vi "Test Broadcast Seen from Process Added Before Attaching to Owning Application.vi"(8 "error in (no error)":errorcluster, 11 "Test Case In":refnum<class "Monitor Broadcasts Test.lvclass">) -> (0 "error out":errorcluster, 3 "Test Case Out":refnum<class "Monitor Broadcasts Test.lvclass">)   [LabVIEW 2020, in "Monitor Broadcasts Test.lvclass"]
uses:
  Monitor Broadcasts Test.lvclass
  C:/Program Files (x86)/National Instruments/LabVIEW 2020/vi.lib/Astemes/LUnit/Test Case.lvclass
  source/Broadcast Message Receiver/Broadcast Message Receiver.lvclass
  C:/Git/astemes-triarc-debugger/source/Process/Debug Process.lvclass
  <vilib>/Astemes/Triarc Framework/Application/Application.lvclass
  C:/Program Files (x86)/National Instruments/LabVIEW 2020/vi.lib/Astemes/Triarc Framework/Process/Process.lvclass
  <vilib>/Astemes/Triarc Framework/Process/Process.lvclass
  <vilib>/Astemes/Triarc Framework/Process/Process.lvclass/Process.ctl
  <vilib>/Astemes/Triarc Framework/Application/Application.lvclass/Application.ctl
  source/Process/Debug Process.lvclass/Debug Process.ctl
  source/Broadcast Message Receiver/Broadcast Message Receiver.lvclass/Broadcast Message Receiver.ctl
  <vilib>/Astemes/LUnit/Test Case.lvclass/Test Case.ctl
  322eb4a3-86ea-404a-b8c1-ce150151c392.vi
  64c6a37a-23a3-4de3-a18c-a5f87f217a42.vi
  01074fa8-ee8a-411d-bc8b-fc92c4f90959.vi
  <vilib>/Astemes/Triarc Framework/Application/Private/Add Process to Map.vi
  <vilib>/Astemes/Triarc Framework/Application/Private/Throw Error If Process Already in App.vi
  <vilib>/Astemes/Triarc Framework/Process/Protected/Messaging/Send Message.vi
  <vilib>/Astemes/Triarc Framework/Process/Public/Lifecycle/Get Lifecycle State.vi
  <vilib>/Astemes/Triarc Framework/Process/Protected/SubVIs/Set Context.vi
  source/Process/Public/Lifecycle/Get Lifecycle State.vi
  source/Process/Protected/Messaging/Enqueue Message.vi
  source/Process/Private/SubVIs/Wait for finish.vi
  source/Process/Private/SubVIs/Set Lifecycle State.vi
  <vilib>/Astemes/Triarc Framework/Process/Private/SubVIs/Wait for finish.vi
  <vilib>/Astemes/Triarc Framework/Process/Private/SubVIs/Set Lifecycle State.vi
  <vilib>/Astemes/LUnit/Palette/Pass.vi
  <vilib>/Astemes/LUnit/Palette/Fail.vi
  <vilib>/Astemes/LUnit/Compare Variants.vi
  <vilib>/Astemes/LUnit/Describe Comparison.vi
  <vilib>/Astemes/LUnit/Set Assertion Type.vi
  <vilib>/Astemes/Triarc Framework/Application/Public/Get Process.vi
  <vilib>/Astemes/Triarc Framework/Process/Private/SubVIs/Handle Debug Data.vi
  <vilib>/Utility/error.llb/Clear Errors.vi
  <vilib>/Astemes/Triarc Framework/Process/Public/Lifecycle/Leave Process Loop.vi
  <vilib>/Astemes/LUnit/Add test result.vi
  <vilib>/Astemes/LUnit/Variant to string.vi
  <vilib>/Astemes/Triarc Framework/Application/Private/Retrieve Process from App.vi
  <vilib>/Astemes/Triarc Framework/Application/Private/Parse Process Name.vi
  <vilib>/Astemes/Triarc Framework/Application/Private/Get Process from Map.vi
  <vilib>/Astemes/Triarc Framework/Logging/Log Debug.vi
  <vilib>/AdvancedString/1D String Array to Delimited String.vi
  <vilib>/Utility/High Resolution Relative Seconds.vi
  <vilib>/Astemes/LUnit/LUnit Record Assertion Result.vi
  <vilib>/Astemes/Triarc Framework/Process/Protected/Messaging/Request Message.vi
  <vilib>/AdvancedString/Delimited String to 1D String Array.vi
  <vilib>/Astemes/LUnit/LUnit Aggregate Assertion Results.vi
  <vilib>/Astemes/Triarc Framework/Process/Private/SubVIs/Enqueue Request Message.vi
  <vilib>/Astemes/LUnit/Method Result/LUnit Merge Status.vi
  <vilib>/Astemes/LUnit/LUnit Concatenate result strings.vi
  source/Mock Data Listener/Mock Data Listener.lvclass
  C:/Git/astemes-triarc-debugger/source/Debug Data Event/Debug Data Listener.lvclass
  <vilib>/Utility/error.llb/Error Cluster From Error Code.vi
  <vilib>/Astemes/Triarc Framework/Process/Public/Read Name.vi
  <vilib>/Astemes/Triarc Framework/Process/Private/SubVIs/Wait for Response Message.vi
  <vilib>/Utility/Data Type/Get Type Information.vi
  <vilib>/Utility/LVClass/Get LV Class Name.vi
  source/Process/Debug Process.lvclass
panel:
  out "x+1":i32
  out "Count":i32
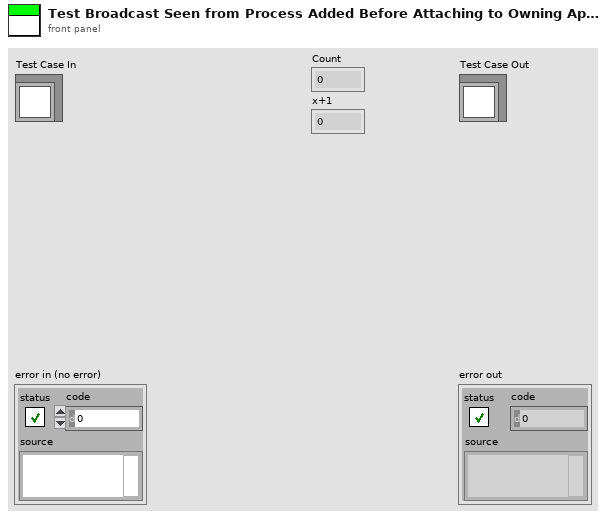
[diagram p1: front panel]
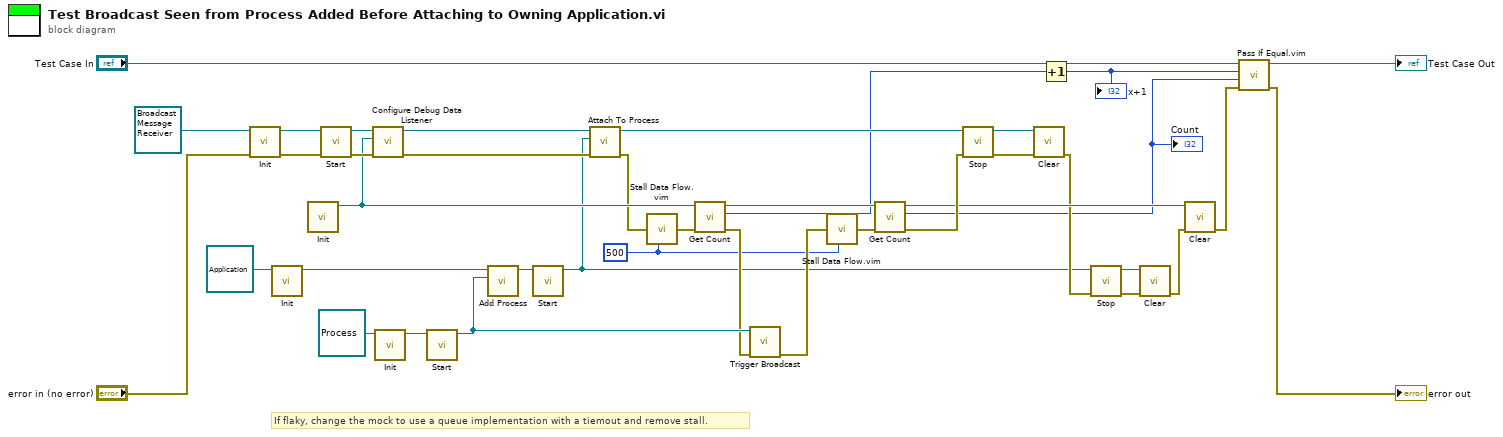
[diagram p0: block diagram]
diagram:
  w1 = u32 500 ("milliseconds to wait")
  # "If flaky, change the mock to use a queue implementation with a tiemout and remove stall."
  n1 = call-dynamic "Init.vi"("error in (no error)"="error in (no error)", "Process In"=refnum<class "Broadcast Message Receiver.lvclass"> refnum ("Broadcast Message Receiver.lvclass")) -> ("error out"=w34:errorcluster, "Process Out"=w35:refnum<class "Broadcast Message Receiver.lvclass">)  [unwired: 8 in]
  n2 = call-dynamic "Init.vi"("Process In"=refnum<class "Application.lvclass"> refnum ("Application In")) -> ("Process Out"=w24:refnum<class "Application.lvclass">)  [unwired: 9 in, 1 out]
  n3 = call "Init.vi"() -> ("Mock Data Listener Out"=w23:refnum<class "Mock Data Listener.lvclass">)  [unwired: 10 in, 1 out]
  n4 = call <vilib>:"Start.vi"("error in (no error)"=w34, "Process In"=w35) -> ("error out"=w32:errorcluster, "Process Out"=w33:refnum<class "Broadcast Message Receiver.lvclass">)  [unwired: 7 in, 1 out]
  n5 = call "Configure Debug Data Listener.vi"("error in (no error)"=w32, "Debug Data Listener"=w23, "Debug Message Receiver In"=w33) -> ("error out"=w6:errorcluster, "Debug Message Receiver Out"=w31:refnum<class "Broadcast Message Receiver.lvclass">)  [unwired: 7 in]
  n6 = call-dynamic "Init.vi"("Process In"=refnum<class "Process.lvclass"> refnum) -> ("Process Out"=w26:refnum<class "Process.lvclass">)  [unwired: 9 in, 1 out]
  n7 = call <vilib>:"Start.vi"("Process In"=w26) -> ("Process Out"=w20:refnum<class "Process.lvclass">)  [unwired: 8 in, 2 out]
  n8 = call <vilib>:"Add Process.vi"("Process"=w20, "Application In"=w24) -> ("Application Out"=w7:refnum<class "Application.lvclass">)  [unwired: 8 in, 1 out]
  n9 = call <vilib>:"Start.vi"("Process In"=w7) -> ("Process Out"=w4:refnum<class "Application.lvclass">)  [unwired: 8 in, 2 out]
  n10 = call "Attach To Process.vi"("error in (no error)"=w6, "Process In"=w4, "Broadcast Message Receiver In"=w31) -> ("error out"=w5:errorcluster, "Broadcast Message Receiver Out"=w30:refnum<class "Broadcast Message Receiver.lvclass">)  [unwired: 7 in]
  n11 = call "Stall Data Flow.vim"("value in"=w5, "milliseconds to wait"=w1) -> ("value out"=w3:errorcluster)  [unwired: 1 out]
  n12 = call "Get Count.vi"("error in (no error)"=w3, "Mock Data Listener In"=w23) -> ("error out"=w19:errorcluster, "Count"=w10:i32, "Mock Data Listener Out"=w22:refnum<class "Mock Data Listener.lvclass">)  [unwired: 7 in]
  n13 = call <vilib>:"Trigger Broadcast.vi"("error in (no error)"=w19, "Process in"=w20) -> ("error out"=w18:errorcluster)  [unwired: 8 in, 1 out]
  n14 = call "Stall Data Flow.vim"("value in"=w18, "milliseconds to wait"=w1) -> ("value out"=w2:errorcluster)  [unwired: 1 out]
  n15 = call "Get Count.vi"("error in (no error)"=w2, "Mock Data Listener In"=w22) -> ("error out"=w21:errorcluster, "Count"=w8:i32, "Mock Data Listener Out"=w14:refnum<class "Mock Data Listener.lvclass">)  [unwired: 7 in]
  "Count" <- w8
  n16 = call <vilib>:"Stop.vi"("error in (no error)"=w21, "Process In"=w30) -> ("error out"=w28:errorcluster, "Process Out"=w29:refnum<class "Broadcast Message Receiver.lvclass">)  [unwired: 7 in, 1 out]
  n17 = call-dynamic "Clear.vi"("error in (no error)"=w28, "Process In"=w29) -> ("error out"=w12:errorcluster)  [unwired: 9 in]
  n18 = Increment(x=w10) -> (x+1=w9:i32)
  "x+1" <- w9
  n19 = call <vilib>:"Stop.vi"("error in (no error)"=w12, "Process In"=w4) -> ("error out"=w15:errorcluster, "Process Out"=w16:refnum<class "Application.lvclass">)  [unwired: 7 in, 1 out]
  n20 = call-dynamic "Clear.vi"("error in (no error)"=w15, "Application In"=w16) -> ("error out"=w13:errorcluster)  [unwired: 9 in]
  n21 = call "Clear.vi"("error in (no error)"=w13, "Mock Data Listener in"=w14) -> ("error out"=w11:errorcluster)  [unwired: 9 in]
  n22 = call "Pass If Equal.vim"("error in (no error)"=w11, "Actual"=w8, "Expected"=w9, "LUnit Test Case In"="Test Case In") -> ("error out"=→"error out":errorcluster, "LUnit Test Case Out"=→"Test Case Out":refnum<class "Monitor Broadcasts Test.lvclass">)  [unwired: 6 in]
